vi "提取子数组.vi"() -> ()   [LabVIEW 2010]
panel:
  out "子数组":dbl[][](array[numeric]) format="%.2f"
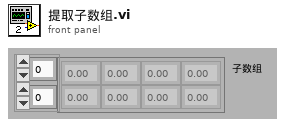
[diagram p1: front panel]
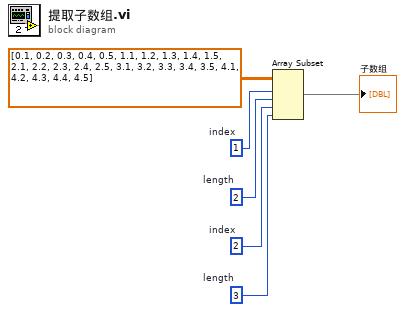
[diagram p0: block diagram]
diagram:
  w1 = 3  # length
  w2 = 2  # index
  w3 = 2  # length
  w4 = 1  # index
  n1 = Array Subset "Array Subset"(array=dbl[][] [[0.1, 0.2, 0.3, 0.4, 0.5], [1.1, 1.2, 1.3, 1.4, 1.5], [2.1, 2.2, 2.3, 2.4, 2.5], [3.1, 3.2, 3.3, 3.4, 3.5], [4.1, 4.2, 4.3, 4.4, 4.5]], index (row)=w4, length (row)=w3, index (col)=w2, length (col)=w1) -> (→"子数组":dbl[][])
